vi "sub_log_basic.vi"(8 "error in":errorcluster, 10 "desc":string, 11 "Title":string) -> (0 "error out":errorcluster)   [LabVIEW 2019]
uses:
  _ctrl/rw.ctl
  _ctrl/create-rw-close.ctl
  Data Process/type-data.ctl
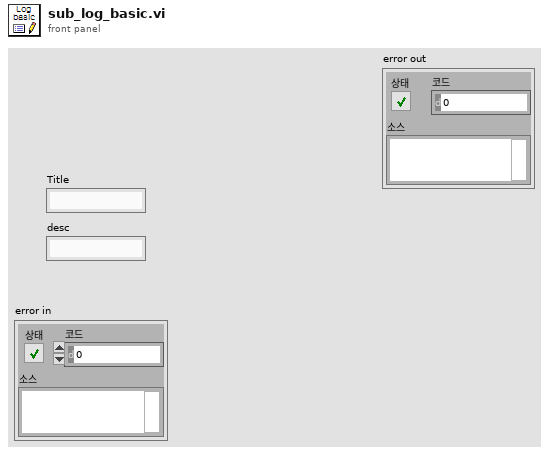
[diagram p1: front panel]
types:
  T1 = typedef "type-data.ctl" = cluster{"dup path":path, "data":string}
  T2 = typedef "create-rw-close.ctl" = enum16{"create", "write", "read", "delete", "close"}
  T3 = typedef "rw.ctl" = enum16{"read", "write"}
  T4 = typedef "config_aging.ctl" = cluster{"Setting":T5, "TestName":string, "Result path":path, "파일 생성 주기[N]":u8, "Test Specs":T6}
  T5 = typedef "Setting_reg.ctl" = cluster{"제어 전압[V]":dbl, "출력전압[V]":dbl, "전류[A]":dbl, "출력전류[A]":dbl, "ON[초]":dbl, "OFF[초]":dbl, "Irms 허용치 from ":dbl, "Irms 허용치 to":dbl, "AO Delay ms":u32, "Log":path, "result":path}
  T6 = typedef "Breakdown-Spec.ctl" = cluster{"제어단 단선 Irms[mA](이하)":dbl, "제어단 특성 전류 Irms[mA] Max":dbl, "제어단 특성 전류 Irms[mA] Min":dbl, "출력단 단선 Irms[mA](이하)":dbl, "출력단 특성 전류 Irms[mA]  Max":dbl, "출력단 특성전류 Irms[mA]  Min":dbl, "온도[degree]":dbl}
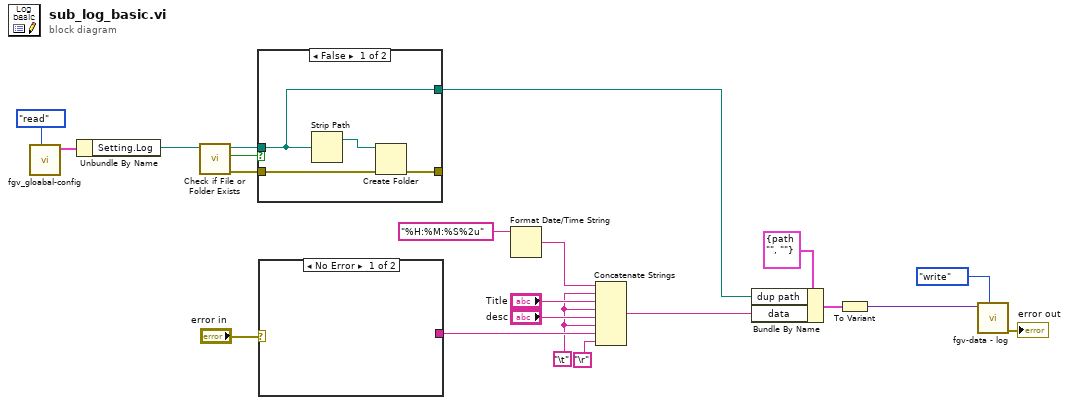
[diagram p0: block diagram]
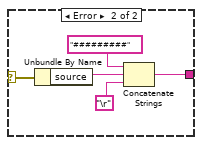
[diagram p2: hidden frame]
diagram:
  w15 = "\t"
  n1 = call "fgv_gloabal-config.vi"("cmd"=rw."read") -> ("config_aging 2"=w9:T4)  [unwired: 10 in]
  n2 = Unbundle By Name(w9) -> ("Setting.Log"=w8:path)
  n3 = call <vilib>:"Check if File or Folder Exists.vi"("path"=w8) -> ("error out"=w11:errorcluster, "file or folder exists?"=w12:bool, "dup path"=w21:path)  [unwired: 8 in]
  n4 = case shown="False" w12 {
    tunnel: w21 -> [w23 w27]
    tunnel: [w23 w27] -> w2
    tunnel: w11 -> [w25 w26]
    tunnel: [w24 w26] -> _
    frame False {
      n5 = Strip Path(path=w23) -> (stripped path=w22:path)  [unwired: 1 out]
      n6 = Create Folder(path (use dialog)=w22, error in=w25) -> (error out=w24:errorcluster)  [unwired: 1 in, 2 out]
    }
    frame True {
    }
  }
  n7 = case shown="No Error" "error in" {
    selector: "error in" -> [_ w32]
    tunnel: [_ w28] -> w16
    frame No Error {
    }
    frame Error {
      n8 = Unbundle By Name(w32) -> ("source"=w30:string)
      n9 = Concatenate Strings("#########" ("문자열"), w30, "\r") -> (w28:string)
    }
  }
  n10 = Format Date/Time String(time format string (%c)="%H:%M:%S%2u" ("시간 포맷 문자열 (%c)")) -> (date/time string=w19:string)  [unwired: 2 in]
  n11 = Concatenate Strings(w19, w15, "Title", w15, "desc", w15, w16, "\r") -> (w5:string)
  n12 = Bundle By Name(cluster=T1 {"dup path"=path "", "data"=""}, "dup path"=w2, "data"=w5) -> (w4:T1)
  n13 = To Variant(anything=w4) -> (Variant=w3:variant)
  n14 = call "fgv-data - log.vi"("cmd"=create-rw-close."write", "element"=w3) -> ("error out"=→"error out":errorcluster)  [unwired: 8 in, 1 out]
